vi "_PC_RTFunc_AccessExtDI.vi"(7 "Function":enum16{"Init", "Write", "Read"}(ring)=enum."Write", 8 "error in (no error)":errorcluster, 10 "DI in":T1=[{"Label"="", "Boolean"=FALSE}, {"Label"="", "Boolean"=FALSE}, {"Label"="", "Boolean"=FALSE}, {"Label"="", "Boolean"=FALSE}, {"Label"="", "Boolean"=FALSE}, {"Label"="", "Boolean"=FALSE}, {"Label"="", "Boolean"=FALSE}, {"Label"="", "Boolean"=FALSE}]) -> (0 "error out":errorcluster, 2 "DI out":cluster{"Label":string, "Boolean":bool}[](array[cluster]))   [LabVIEW 2018]
uses:
  RT/PublicSubVI/Ctl/_ctl_RT_extDO.ctl
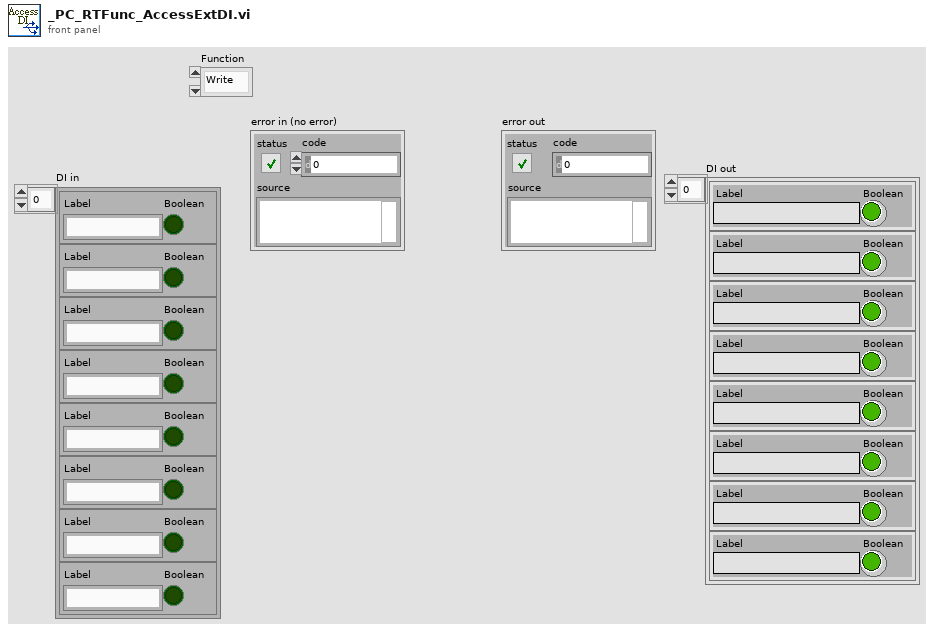
[diagram p1: front panel]
types:
  T1 = typedef "_ctl_RT_extDO.ctl" = cluster{"Label":string, "Boolean":bool}[]
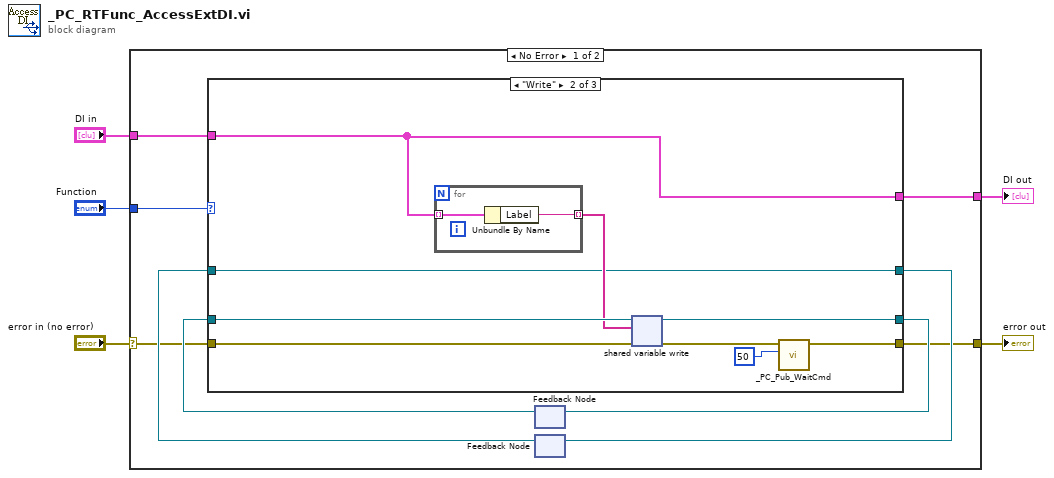
[diagram p0: block diagram]
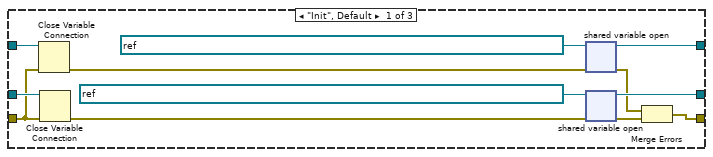
[diagram p2: hidden frame]
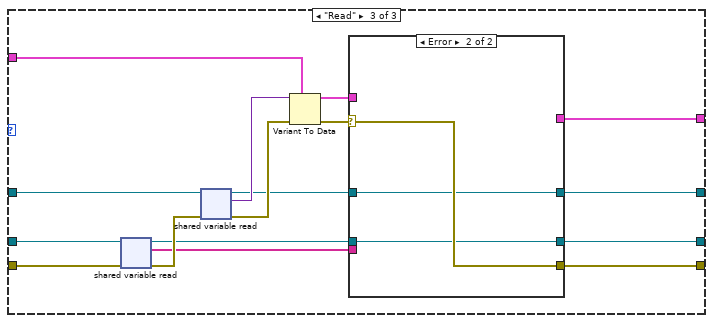
[diagram p3: hidden frame]
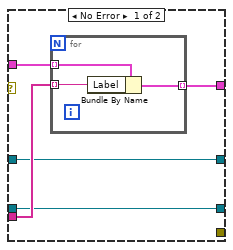
[diagram p4: hidden frame]
diagram:
  n1 = case shown="No Error" "error in (no error)" {
    selector: "error in (no error)" -> [w9 w66]
    tunnel: [w10 w66] -> w5
    tunnel: "DI in" -> [w8 w65]
    tunnel: "Function" -> [w7 _]
    tunnel: [w6 w65] -> w1
    frame No Error {
      n2 = feedback #1() -> (w13:refnum<k21>)  [unwired: 1 in]
      n3 = feedback #2() -> (w11:refnum<k21>)  [unwired: 1 in]
      n4 = case shown="\"Write\"" w7 {
        tunnel: w13 -> [w19 w35 w53]
        tunnel: [w25 w34 w42] -> w14
        tunnel: w11 -> [w18 w31 w51]
        tunnel: [w23 w31 w44] -> w12
        tunnel: w8 -> [_ w30 w48]
        tunnel: [w20 w27 w45] -> w10
        tunnel: w9 -> [w17 w32 w52]
        tunnel: [_ w30 w38] -> w6
        frame "Init", Default {
          n5 = Close Variable Connection(8:w17, 11:w18) -> (0:w16:errorcluster)
          n6 = Close Variable Connection(8:w17, 11:w19) -> (0:w15:errorcluster)
          n7 = shared-variable-open(refnum<k21> "ni.var.psp://NI-sbRIO/_RT_CtrlLoop_DigitalAnalogueInput_Variables/ExtDI" ("shared variable refnum in"), w16) -> (w23:refnum<k21>, w22:errorcluster)
          n8 = shared-variable-open(refnum<k21> "ni.var.psp://NI-sbRIO/_RT_CtrlLoop_DigitalAnalogueInput_Variables/ExtDI_Labels" ("shared variable refnum in"), w15) -> (w25:refnum<k21>, w21:errorcluster)
          n9 = Merge Errors(w22, w21) -> (w20:errorcluster)
        }
        frame "Write" {
          n10 = for {
            tunnel: w30 -> [w37] mode=indexing
            tunnel: [w36] -> w33 mode=indexing
            n11 = Unbundle By Name(w37) -> ("Label"=w36:string)
          }
          n12 = shared-variable-write(w35, w32, w33) -> (w34:refnum<k21>, w28:errorcluster)
          n13 = call "_PC_Pub_WaitCmd.vi"("milliseconds to wait"=u32 50, "error in (no error)"=w28) -> ("error out"=w27:errorcluster)  [unwired: 9 in]
        }
        frame "Read" {
          n14 = shared-variable-read(w53, w52) -> (w41:refnum<k21>, w50:errorcluster, w40:string[])
          n15 = shared-variable-read(w51, w50) -> (w43:refnum<k21>, w49:errorcluster, w47:variant)
          n16 = Variant To Data(error in=w49, type=w48, Variant=w47) -> (data=w39:T1, error out=w46:errorcluster)
          n17 = case shown="Error" w46 {
            selector: w46 -> [_ w64]
            tunnel: [_ w64] -> w45
            tunnel: [w56 w63] -> w44
            tunnel: w43 -> [w56 w63]
            tunnel: [w54 w62] -> w42
            tunnel: w41 -> [w54 w62]
            tunnel: w40 -> [w57 _]
            tunnel: w39 -> [w58 _]
            tunnel: [w55 _] -> w38
            frame No Error {
              n18 = for {
                tunnel: w58 -> [w61] mode=indexing
                tunnel: w57 -> [w60] mode=indexing
                tunnel: [w59] -> w55 mode=indexing
                n19 = Bundle By Name(cluster=w61, "Label"=w60) -> (w59:cluster{"Label":string, "Boolean":bool})
              }
            }
            frame Error {
            }
          }
        }
      }
      n20 = feedback-in #1(w14) -> ()
      n21 = feedback-in #2(w12) -> ()
    }
    frame Error {
    }
  }
  "error out" <- w5
  "DI out" <- w1
